vi "Global 1.vi"() -> ()   [LabVIEW 2016]
uses:
  ElectrometerError/Controls/errorType.ctl
  ElectrometerError/ElectrometerError.lvclass
panel:
  out "ErrorArray":T1[](array[typedef])
  in  "errorLog":string
  in  "Range":dbl=20.0
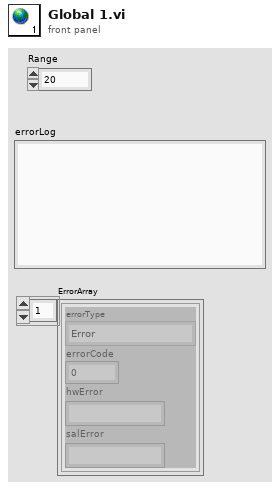
[diagram p1: front panel]
types:
  T1 = typedef "ElectrometerError.lvclass/errorType.ctl" = cluster{"errorType":enum16{"Error", "Warning", "None"}, "errorCode":dbl, "hwError":string, "salError":string}
diagram:
